vi "Main_Litho_driver.vi"() -> ()   [LabVIEW 2016]
uses:
  litho folder/Global/Lithography Data.vi
panel:
  in  "Application":refnum<k7>
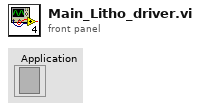
[diagram p1: front panel]
types:
  T1 = cluster{"Name":string, "Litho":cluster{"X":dbl, "Y":dbl, "Speed":dbl, "Voltage":dbl}[]}[]
  T2 = typedef "References.ctl" = cluster{"Zcontroller":refnum<k7>, "Litho":refnum<k7>, "Scan":refnum<k7>, "SignalIO":refnum<k7>, "Application":refnum<k7>}
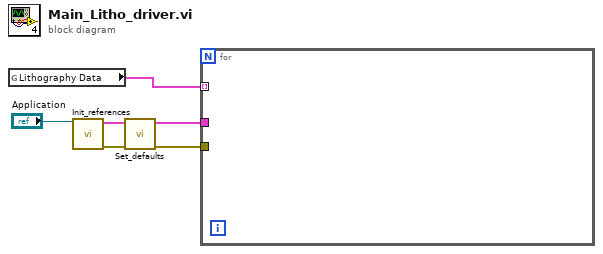
[diagram p0: block diagram]
diagram:
  n1 = global read "Lithography Data.vi" "Lithography Data"() -> (w1:T1)
  n2 = call "Init_references.vi"("Application"="Application") -> ("error out"=w6:errorcluster, "References"=w2:T2)  [unwired: 9 in]
  n3 = call "Set_defaults.vi"("error in"=w6, "References In"=w2) -> ("error out"=w4:errorcluster, "References Out"=w3:T2)  [unwired: 8 in]
  n4 = for {
    tunnel: w4 -> [_]
    tunnel: w3 -> [_]
    tunnel: w1 -> [_] mode=indexing
  }
